vi "Write Plot Array.vi"(8 "error in (no error)":errorcluster, 9 "Plot Property Array":T1=[{"Bar Plot Style"=0, "DigitalLineStyle"=1, "TransitionLocation"=2, "Transition Type"=0, "Fill To"=-1, "Fill/Pt. Color"=16448250, "Label Style"=3, "Line Style"=0, "Line Width"=0, "Plot Color"=16448250, "Plot Interpolation"=2, "Plot Name"="Plot 0", "Point Style"=1, "Visible?"=TRUE, "XScaleIdx"=0, "YScaleIdx"=0}, {"Bar Plot Style"=0, "DigitalLineStyle"=1, "TransitionLocation"=2, "Transition Type"=0, "Fill To"=-1, "Fill/Pt. Color"=16448250, "Label Style"=3, "Line Style"=0, "Line Width"=0, "Plot Color"=16448250, "Plot Interpolation"=2, "Plot Name"="Plot 1", "Point Style"=1, "Visible?"=TRUE, "XScaleIdx"=0, "YScaleIdx"=0}], 11 "2D Feather.lvclass in":refnum<class "2D Feather.lvclass">) -> (0 "error out":errorcluster, 3 "2D Feather.lvclass out":refnum<class "2D Feather.lvclass">)   [LabVIEW 2020, in "2D Feather.lvclass"]
uses:
  <vilib>/Math Plots/2D Math Plots/2D Feather/2D Feather/2D Feather.lvclass
  <vilib>/Math Plots/2D Math Plots/2D Plot/2D Plot/Typedef/Plot Property Array.ctl
  <vilib>/Math Plots/2D Math Plots/2D Plot/2D Plot/Typedef/Plot Property.ctl
  <vilib>/Math Plots/2D Math Plots/2D Feather/2D Feather/2D Feather.lvclass/2D Feather.ctl
  <vilib>/Math Plots/2D Math Plots/2D Plot/2D Plot/2D Plot.lvclass
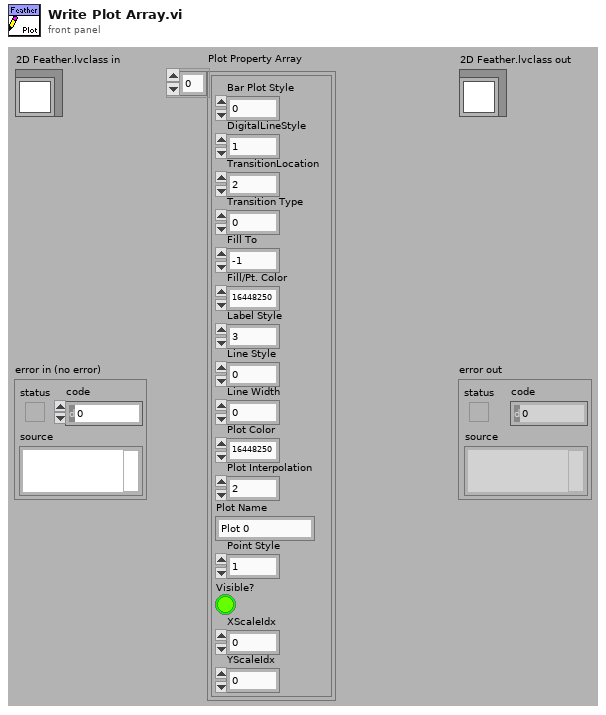
[diagram p1: front panel]
types:
  T1 = typedef "2D Plot.lvclass/Plot Property Array.ctl" = T2[]
  T2 = typedef "2D Plot.lvclass/Plot Property.ctl" = cluster{"Bar Plot Style":u8, "DigitalLineStyle":u8, "TransitionLocation":u8, "Transition Type":u8, "Fill To":i16, "Fill/Pt. Color":u32, "Label Style":u8, "Line Style":u8, "Line Width":u8, "Plot Color":u32, "Plot Interpolation":u8, "Plot Name":string, "Point Style":u8, "Visible?":bool, "XScaleIdx":u32, "YScaleIdx":u32}
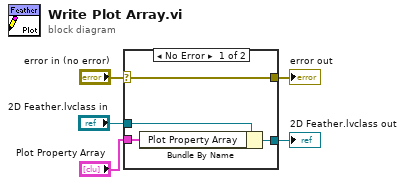
[diagram p0: block diagram]
diagram:
  n1 = case shown="No Error" "error in (no error)" {
    selector: "error in (no error)" -> [w9 w10]
    tunnel: [w9 w10] -> w4
    tunnel: [w7 w11] -> w2
    tunnel: "2D Feather.lvclass in" -> [w8 w11]
    tunnel: "Plot Property Array" -> [w6 _]
    frame No Error {
      n2 = Bundle By Name(cluster=w8, "Plot Property Array"=w6) -> (w7:refnum<class "2D Feather.lvclass">)
    }
    frame Error {
    }
  }
  "error out" <- w4
  "2D Feather.lvclass out" <- w2
